vi "Convert Resistance to Temperature.vi"(8 "error in (no error)":errorcluster, 11 "Resistance (Ohms)":dbl=10000.0) -> (0 "error out":errorcluster, 3 "Temperature (C)":dbl)   [LabVIEW 2025, in "Submodule EOL.lvlib" / "Submodule EOL.lvclass"]
uses:
  Submodule EOL.lvclass
  Submodule EOL.lvclass/Submodule EOL.ctl
panel:
  # "Murata Thermistor NXFT15XH103FEAB045"
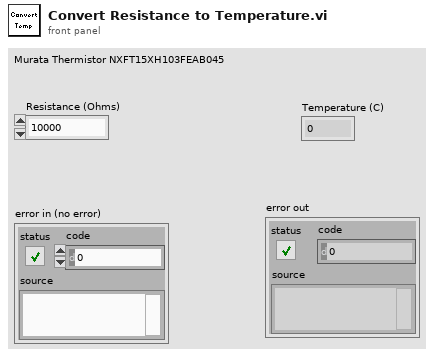
[diagram p1: front panel]
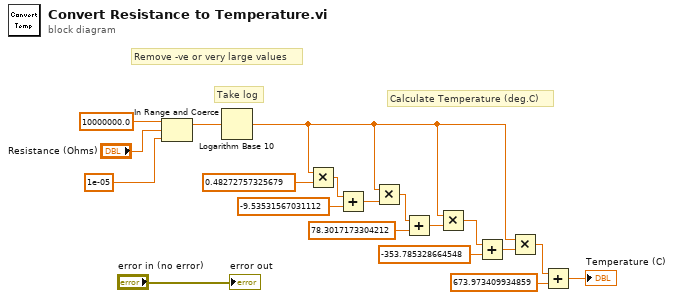
[diagram p0: block diagram]
diagram:
  # "Calculate Temperature (deg.C)"
  # "Take log"
  # "Remove -ve or very large values"
  n1 = In Range and Coerce(upper limit=10000000.0, x="Resistance (Ohms)", lower limit=1e-05) -> (coerced(x)=w18:dbl)  [unwired: 1 out]
  n2 = Logarithm Base 10(1:w18) -> (0:w4:dbl)
  n3 = Multiply(x=w4, y=0.48272757325679 ("Coefficient")) -> (x*y=w15:dbl)
  n4 = Add(x=w15, y=-9.53531567031112 ("Coefficient")) -> (x+y=w11:dbl)
  n5 = Multiply(x=w4, y=w11) -> (x*y=w12:dbl)
  n6 = Add(x=w12, y=78.3017173304212 ("Coefficient")) -> (x+y=w8:dbl)
  n7 = Multiply(x=w4, y=w8) -> (x*y=w9:dbl)
  n8 = Add(x=w9, y=-353.785328664548 ("Coefficient")) -> (x+y=w5:dbl)
  n9 = Multiply(x=w4, y=w5) -> (x*y=w6:dbl)
  n10 = Add(x=w6, y=673.973409934859 ("Coefficient")) -> (x+y=→"Temperature (C)":dbl)
  "error out" <- "error in (no error)"
